vi "acquire_FGV.vi"(7 "Mode":T1, 8 "error in":errorcluster, 11 "Parameter in":variant) -> (0 "error out":errorcluster, 3 "Parameter out":variant)   [LabVIEW 2016]
uses:
  Tools/three_modes.ctl
  MainFGV/cluster_main_FGV.ctl
  Config/Channel_config.ctl
  Config/test_config.ctl
  Config/feedType.ctl
  <vilib>/DAQmx/read.llb/DAQmx Read (Analog 2D DBL NChan NSamp).vi
  <vilib>/Analysis/baseanly.llb/Mean (DBL).vi
  <vilib>/DAQmx/miscellaneous.llb/DAQmx Fill In Error Info.vi
  <vilib>/Analysis/NI_AALBase.lvlib
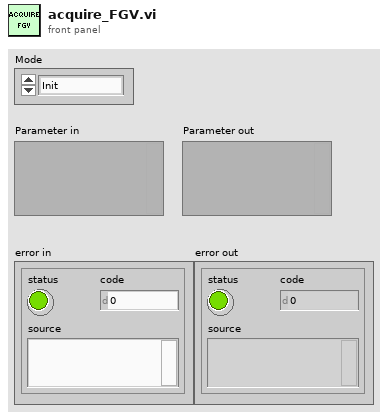
[diagram p1: front panel]
types:
  T1 = typedef "three_modes.ctl" = enum16{"Init", "Exec", "End"}
  T2 = typedef "cluster_main_FGV.ctl" = cluster{"Simulation?":bool, "ChanConfigs":T3[], "Test Config":T4, "Directory":path, "TestName":string, "RawFile":refnum<file>, "InfoFile":refnum<file>, "DataFile":refnum<file>, "task":refnum<k21>, "qRecord":refnum<queue>, "qProcess":refnum<queue>, "feed":T5}
  T3 = typedef "Channel_config.ctl" = cluster{"Canal":i32, "GF":dbl, "SC":bool}
  T4 = typedef "test_config.ctl" = cluster{"HoleDiam":dbl, "MeanLineDiam":dbl, "IncF":dbl, "ElastMod":dbl, "PoissonMod":dbl, "RosType":enum16{"Tipo A", "Tipo B", "Tipo C"}, "Método de análise":enum16{"Não uniforme 2013", "Simplificado 2013", "Simplificado 2008"}, "Pfinal":dbl, "AStop":bool}
  T5 = typedef "feedType.ctl" = enum16{"Manual", "Automático"}
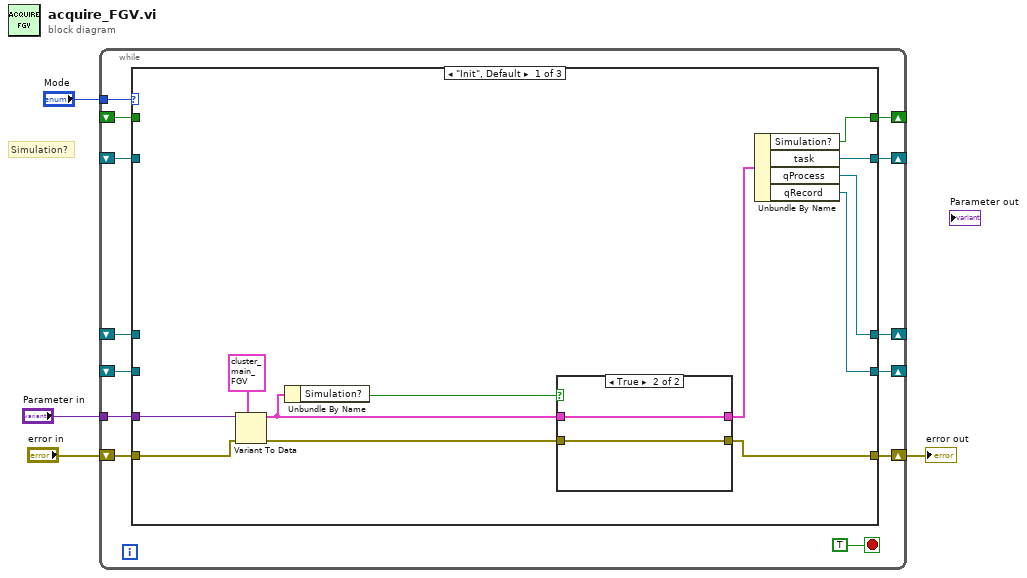
[diagram p0: block diagram]
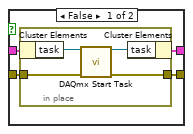
[diagram p2: hidden frame]
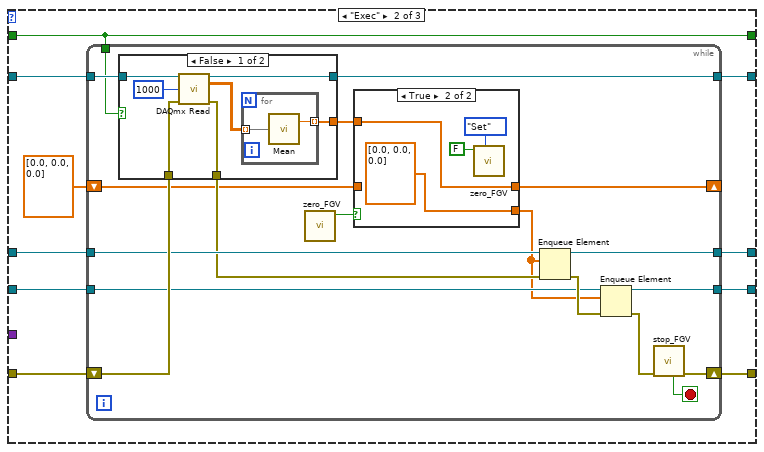
[diagram p3: hidden frame]
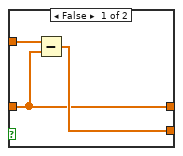
[diagram p4: hidden frame]
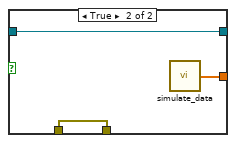
[diagram p5: hidden frame]
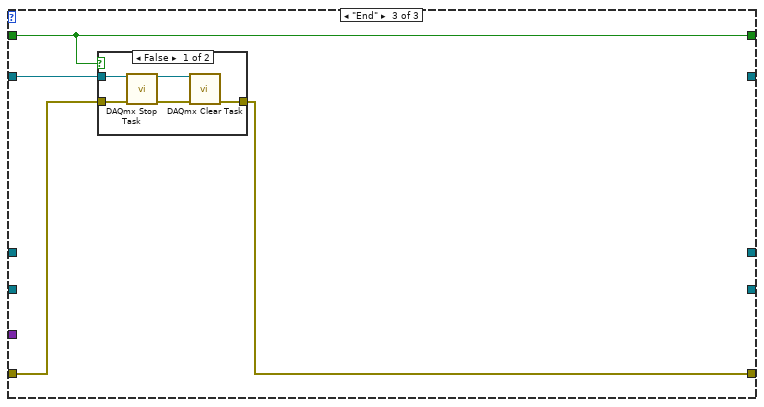
[diagram p6: hidden frame]
diagram:
  # "Simulation?"
  n1 = while {
    tunnel: "Mode" -> [w16]
    tunnel: "Parameter in" -> [w14]
    shift-right: [w12] -> w1
    shift-left: "error in" -> [w15]
    shift-right: [w13] -> _
    shift-left: _ -> [w10]
    shift-right: [w11] -> _
    shift-left: _ -> [w9]
    shift-right: [w8] -> _
    shift-left: _ -> [w7]
    shift-right: [w6] -> _
    shift-left: _ -> [w5]
    stop <- TRUE stop-if-true
    n2 = case shown="\"Init\", Default" w16 {
      tunnel: w15 -> [w27 w49 w88]
      tunnel: w14 -> [w29 _ _]
      tunnel: [w26 w46 _] -> w13
      tunnel: [w22 w48 w87] -> w12
      tunnel: [w25 w44 _] -> w11
      tunnel: w10 -> [_ w47 w90]
      tunnel: w9 -> [_ w45 _]
      tunnel: [w21 w42 _] -> w8
      tunnel: w7 -> [_ w43 _]
      tunnel: [w18 w41 w89] -> w6
      tunnel: w5 -> [_ w41 w89]
      frame "Init", Default {
        n3 = Variant To Data(error in=w27, type=T2 {"Simulation?"=FALSE, "ChanConfigs"=[], "Test Config"={"HoleDiam"=1.4, "MeanLineDiam"=5.0, "IncF"=0.2, "ElastMod"=207.0, "PoissonMod"=0.3, "RosType"=enum."Tipo A", "Método de análise"=enum."Simplificado 2008", "Pfinal"=0.3, "AStop"=TRUE}, "Directory"=path "", "TestName"="", "RawFile"=refnum, "InfoFile"=refnum, "DataFile"=refnum, "task"="", "qRecord"=refnum, "qProcess"=refnum, "feed"=enum."Manual"} ("cluster_main_FGV"), Variant=w29) -> (data=w20:T2, error out=w24:errorcluster)
        n4 = Unbundle By Name(w20) -> ("Simulation?"=w19:bool)
        n5 = case shown="True" w19 {
          tunnel: w24 -> [w33 w38]
          tunnel: [w32 w39] -> w23
          tunnel: [w31 w38] -> w22
          tunnel: w20 -> [w30 w39]
          frame False {
            n6 = in-place {
              in-place-border: w33 -> [w36]
              in-place-border: [w35] -> w31
              n7 = in-place-cluster #1(w30) -> ("task"=w37:refnum<k21>)
              n8 = call <vilib>:"DAQmx Start Task.vi"("task/channels in"=w37, "error in"=w36) -> ("task out"=w34:refnum<k21>, "error out"=w35:errorcluster)  [unwired: 12 in]
              n9 = in-place-cluster #1("task"=w34) -> (w32:T2)
            }
          }
          frame True {
          }
        }
        n10 = Unbundle By Name(w23) -> ("Simulation?"=w18:bool, "task"=w26:refnum<k21>, "qProcess"=w25:refnum<queue>, "qRecord"=w21:refnum<queue>)
      }
      frame "Exec" {
        n11 = while {
          shift-right: [w66] -> w48
          shift-left: w49 -> [w63]
          tunnel: w47 -> [w65]
          tunnel: [w64] -> w46
          tunnel: w45 -> [w62]
          tunnel: [w60] -> w44
          tunnel: w43 -> [w58]
          tunnel: [w57] -> w42
          tunnel: w41 -> [w55]
          shift-right: [w51] -> _
          shift-left: dbl[] [0.0, 0.0, 0.0] ("Dados") -> [w50]
          stop <- w67 stop-if-true
          n12 = case shown="False" w55 {
            tunnel: w65 -> [w81 w85]
            tunnel: [w80 w85] -> w64
            tunnel: w63 -> [w79 w86]
            tunnel: [w77 w86] -> w61
            tunnel: [w75 w84] -> w53
            frame False {
              n13 = call-poly <vilib>:"DAQmx Read.vi"("task/channels in"=w81, "number of samples per channel"=1000, "error in"=w79) -> ("task out"=w80:refnum<k21>, "data"=w76:dbl[][], "error out"=w77:errorcluster)  [unwired: 10 in]
              n14 = for {
                tunnel: w76 -> [w83] mode=indexing
                tunnel: [w82] -> w75 mode=indexing
                n15 = call-poly <vilib>:"Mean.vi"("X"=w83) -> ("mean"=w82:dbl)  [unwired: 1 out]
              }
            }
            frame True {
              n16 = call "simulate_data.vi"() -> ("Dados"=w84:dbl[])
            }
          }
          n17 = call "zero_FGV.vi"() -> ("Zerar?"=w54:bool)  [unwired: 11 in]
          n18 = case shown="True" w54 {
            tunnel: w53 -> [w70 w74]
            tunnel: [w69 dbl[] [0.0, 0.0, 0.0] ("Dados")] -> w52
            tunnel: [w68 w74] -> w51
            tunnel: w50 -> [w68 _]
            frame False {
              n19 = Subtract(x=w70, y=w68) -> (x-y=w69:dbl[])
            }
            frame True {
              n20 = call "zero_FGV.vi"("comandos"=enum16{"Set", "Zerar?"}."Set", "Value"=FALSE) -> ()  [unwired: 9 in, 1 out]
            }
          }
          n21 = Enqueue Element(queue=w62, element=w52, error in (no error)=w61) -> (queue out=w60:refnum<queue>, error out=w59:errorcluster)  [unwired: 1 in, 1 out]
          n22 = Enqueue Element(queue=w58, element=w52, error in (no error)=w59) -> (queue out=w57:refnum<queue>, error out=w56:errorcluster)  [unwired: 1 in, 1 out]
          n23 = call "stop_FGV.vi"("error in (no error)"=w56) -> ("error out"=w66:errorcluster, "parar?"=w67:bool)  [unwired: 9 in]
        }
      }
      frame "End" {
        n24 = case shown="False" w89 {
          tunnel: w90 -> [w95 _]
          tunnel: w88 -> [w94 w96]
          tunnel: [w91 w96] -> w87
          frame False {
            n25 = call <vilib>:"DAQmx Stop Task.vi"("task/channels in"=w95, "error in"=w94) -> ("task out"=w92:refnum<k21>, "error out"=w93:errorcluster)  [unwired: 12 in]
            n26 = call <vilib>:"DAQmx Clear Task.vi"("task in"=w92, "error in"=w93) -> ("error out"=w91:errorcluster)  [unwired: 13 in]
          }
          frame True {
          }
        }
      }
    }
  }
  "error out" <- w1
